vi "MTUchipcorner.vi"(7 "imageParm in":T2, 10 "Image Pixels (U32)":u32[][](array[numeric]), 11 "Param":T1={"Select Mode \n0: Dark\n1: light"=1.0, "Threshold Value"=50.0, "Chip Long Side Size"=25.0, "Chip Long Side Min Tolerance"=0.7, "Chip Long Side Max Tolerance"=1.5, "Chip Short Side Size"=15.0, "Chip Short Side Min Tolerance"=0.7, "Chip Short Side Max Tolerance"=15.0, "Chip Pitch X"=70.0, "Chip Pitch Y"=70.0, "Edge Exclusion Distance"=300.0, "Reserve[11]"=0.0, "Reserve[12]"=0.0, "Parameters[13]"=0.0, "Parameters[14]"=0.0, "Parameters[15]"=0.0, "Parameters[16]"=0.0, "Parameters[17]"=0.0, "Parameters[18]"=0.0, "Parameters[19]"=0.0}) -> (0 "error out":errorcluster, 1 "fPosX":sgl[](array[numeric]), 2 "imageOUT":u32[][](array[numeric]), 3 "boolResult":sgl[](array[numeric]), 4 "fPosY":sgl[](array[numeric]), 5 "fAngle":sgl[](array[numeric]))   [LabVIEW 2017, in "AOILib_MTUchipcorner_V1.lvlib"]
uses:
  <userlib>/AOILib_MTUchipcorner_V1/AOILib_MTUchipcorner_V1.lvlib
  <userlib>/AOILib_MTUchipcorner_V1/AOILib_MTUchipcorner_V1.dll
panel:
  # "綠色: 可能需要經常調整的參數\n灰色: 正常情況下不需要調整的參數\n黃色: 可以提升效率不調整也不會影響的參數"
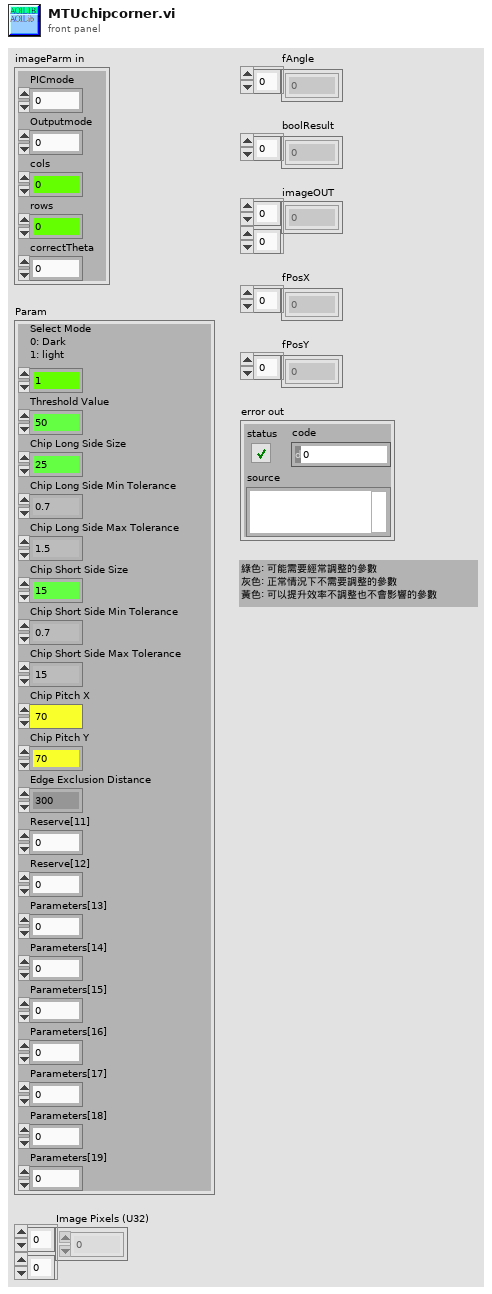
[diagram p1: front panel]
types:
  T1 = cluster{"Select Mode \n0: Dark\n1: light":sgl, "Threshold Value":sgl, "Chip Long Side Size":sgl, "Chip Long Side Min Tolerance":sgl, "Chip Long Side Max Tolerance":sgl, "Chip Short Side Size":sgl, "Chip Short Side Min Tolerance":sgl, "Chip Short Side Max Tolerance":sgl, "Chip Pitch X":sgl, "Chip Pitch Y":sgl, "Edge Exclusion Distance":sgl, "Reserve[11]":sgl, "Reserve[12]":sgl, "Parameters[13]":sgl, "Parameters[14]":sgl, "Parameters[15]":sgl, "Parameters[16]":sgl, "Parameters[17]":sgl, "Parameters[18]":sgl, "Parameters[19]":sgl}
  T2 = cluster{"PICmode":i32, "Outputmode":i32, "cols":i32, "rows":i32, "correctTheta":dbl}
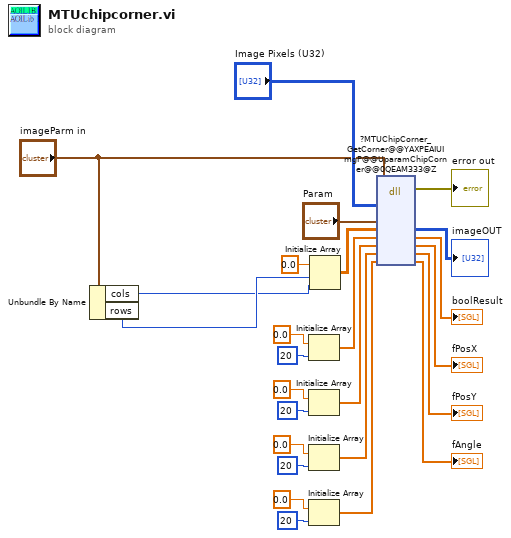
[diagram p0: block diagram]
diagram:
  n1 = Unbundle By Name("imageParm in") -> ("cols"=w1:i32, "rows"=w2:i32)
  n2 = Initialize Array(sgl 0.0 ("element"), 20 ("dimension size")) -> (w5:sgl[])
  n3 = Initialize Array(sgl 0.0 ("element"), 20 ("dimension size")) -> (w9:sgl[])
  n4 = Initialize Array(sgl 0.0 ("element"), 20 ("dimension size")) -> (w13:sgl[])
  n5 = Initialize Array(sgl 0.0 ("element"), 20 ("dimension size")) -> (w17:sgl[])
  n6 = Initialize Array(sgl 0.0 ("element"), w2, w1) -> (w24:sgl[][])
  n7 = dll-call lib="C:/Program Files/National Instruments/LabVIEW 2017/user.lib/AOILib_MTUchipcorner_V1/AOILib_MTUchipcorner_V1.*" fn="?MTUChipCorner_GetCorner@@YAXPEAIUImgP@@UparamChipCorner@@0QEAM333@Z"("imageIN"="Image Pixels (U32)", "imageParm"="imageParm in", "Param"="Param", "imageOUT"=w24, "boolResult"=w5, "fPosX"=w9, "fPosY"=w13, "fAngle"=w17) -> (error out=→"error out":errorcluster, "imageOUT"=→"imageOUT":u32[][], "boolResult"=→"boolResult":sgl[], "fPosX"=→"fPosX":sgl[], "fPosY"=→"fPosY":sgl[], "fAngle"=→"fAngle":sgl[])  [unwired: 7 in, 1 out]
